vi "ChassisDriveDistanceSmart.vi"(8 "Zero":bool, 9 "DriveRight":dbl, 10 "DriveLeft":dbl) -> ()   [LabVIEW 2014, in "ChassisLib.lvlib"]
uses:
  ChassisLib.lvlib
  ChassisRefs.ctl
  <vilib>/addons/control/pid/pid.llb/PID (DBL).vi
  <vilib>/addons/control/pid/NI_PID_pid.lvlib
panel:
  out "Left":cluster{dbl, "PercentComplete":dbl}(graph)
  out "Right":cluster{dbl, "PercentComplete":dbl}(graph)
  out "PercentComplete":dbl format="%#_13g"
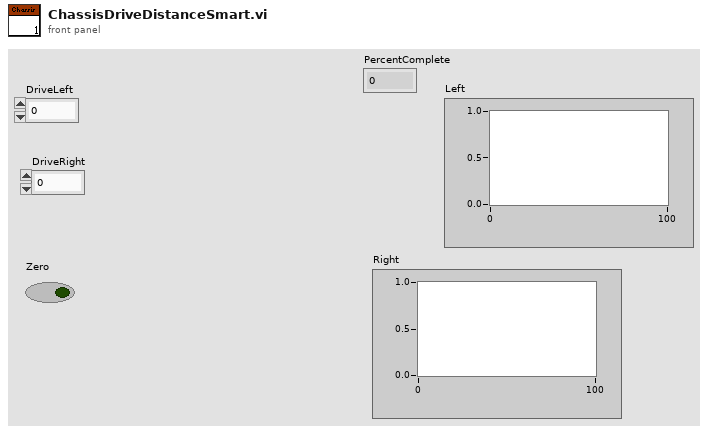
[diagram p1: front panel]
types:
  T1 = typedef "ChassisLib.lvlib/ChassisRefs.ctl" = enum16{"RobotDrive", "Compressor", "DriveEncoderLeft", "DriveEncoderRight", "RioAccel"}
  T2 = typedef "WPI_EncoderDevRef.ctl" = cluster{"DevStatus":errorcluster, "EncoderIndex":T3, "CounterIndex":T4, "DistancePerCount":dbl, "Decoding Type":T5}
  T3 = typedef "FPGA_EncoderIdx.ctl" = enum8{"Enc 0", "Enc 1", "Enc 2", "Enc 3", "Enc 4", "Enc 5", "Enc 6", "Enc 7", "Invalid"}
  T4 = typedef "FPGA_CounterCtrSystemIndex.ctl" = enum8{"Ctr 0", "Ctr 1", "Ctr 2", "Ctr 3", "Ctr 4", "Ctr 5", "Ctr 6", "Ctr 7", "Invalid"}
  T5 = typedef "WPI_EncoderType.ctl" = enum16{"1x", "2x", "4x"}
  T6 = cluster{"proportional gain (Kc)":dbl, "integral time (Ti, min)":dbl, "derivative time (Td, min)":dbl}
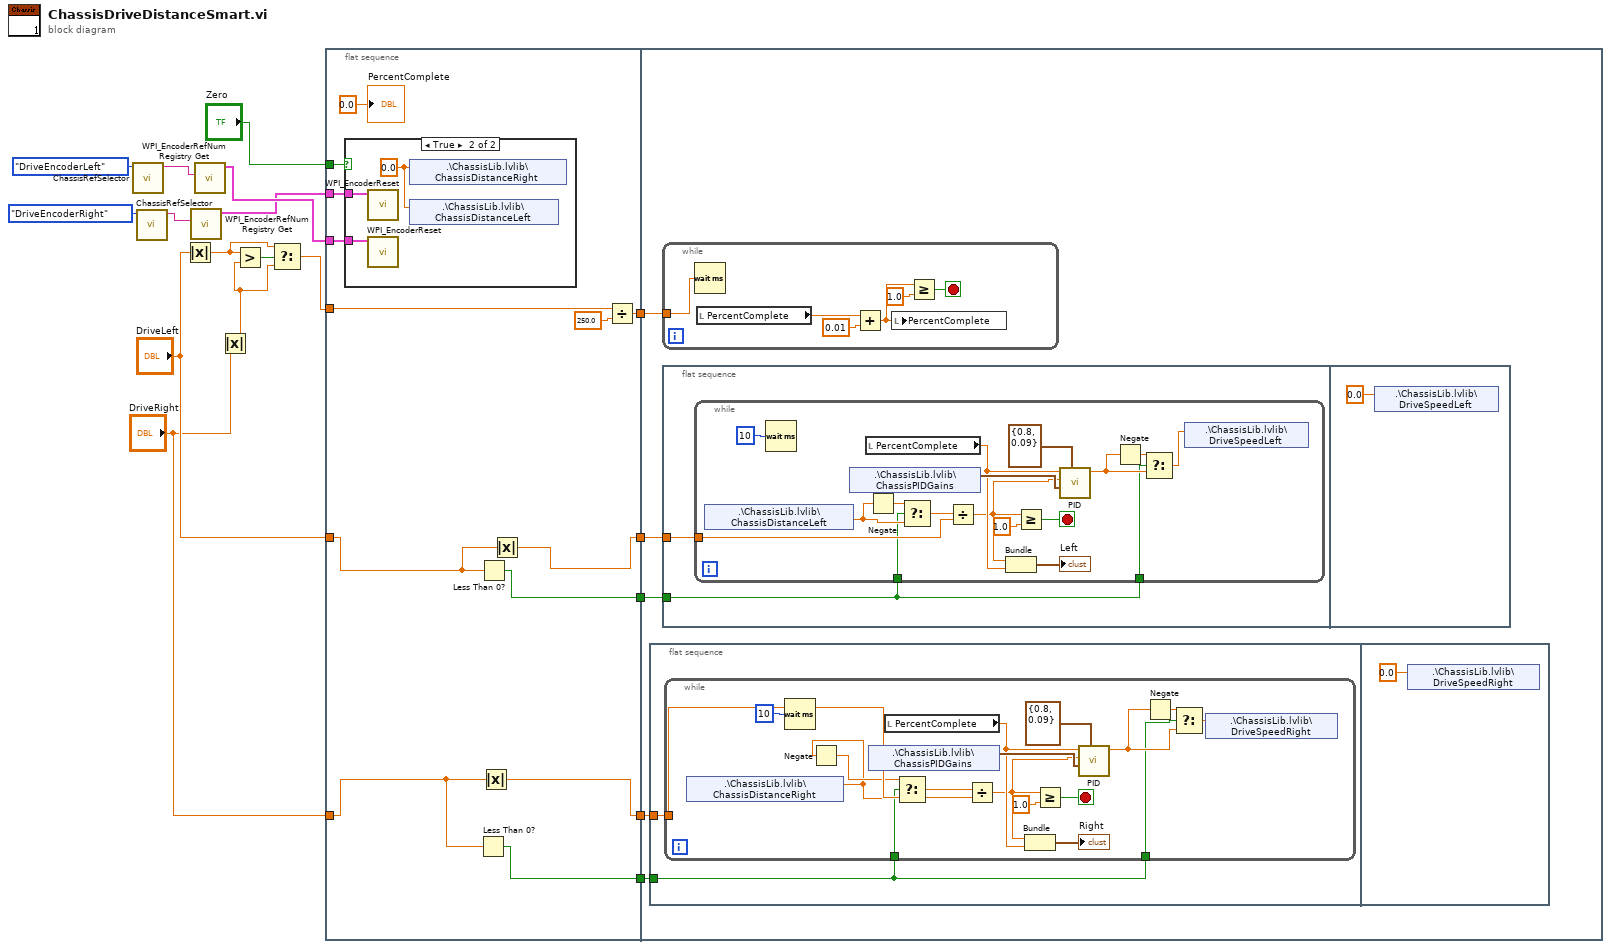
[diagram p0: block diagram]
diagram:
  n1 = call "ChassisRefSelector.vi"("Enum 2"=ChassisRefs."DriveEncoderLeft") -> ("String"=w16:string)  [unwired: 10 in]
  n2 = call "ChassisRefSelector.vi"("Enum 2"=ChassisRefs."DriveEncoderRight") -> ("String"=w15:string)  [unwired: 10 in]
  n3 = Absolute Value(x="DriveLeft") -> (abs(x)=w2:dbl)
  n4 = call <vilib>:"WPI_EncoderRefNum Registry Get.vi"("refnum name"=w15) -> ("EncoderDevRef"=w13:T2)  [unwired: 9 in, 1 out]
  n5 = call <vilib>:"WPI_EncoderRefNum Registry Get.vi"("refnum name"=w16) -> ("EncoderDevRef"=w14:T2)  [unwired: 9 in, 1 out]
  n6 = Absolute Value(x="DriveRight") -> (abs(x)=w1:dbl)
  n7 = Greater?(x=w2, y=w1) -> (0:w12:bool)
  n8 = Select(t=w2, s=w12, f=w1) -> (s? t:f=w11:dbl)
  n9 = flat-sequence {
    tunnel: w14 -> [w31]
    tunnel: w13 -> [w30]
    tunnel: w11 -> [w27]
    tunnel: [w26] -> w10
    tunnel: "DriveLeft" -> [w24]
    tunnel: [w23] -> w8
    tunnel: "DriveRight" -> [w20]
    tunnel: [w21] -> w6
    tunnel: "Zero" -> [w25]
    tunnel: [w22] -> w4
    tunnel: [w19] -> w3
    tunnel: w10 -> [w39]
    tunnel: w8 -> [w38]
    tunnel: w6 -> [w37]
    tunnel: w4 -> [w36]
    tunnel: w3 -> [w35]
    frame #0 {
      n10 = case shown="True" w25 {
        tunnel: w31 -> [_ w34]
        tunnel: w30 -> [_ w33]
        frame False {
        }
        frame True {
          w32 = 0.0 ("ChassisDistanceRight")
          n11 = call <vilib>:"WPI_EncoderReset.vi"("EncoderDevRef"=w33) -> ()  [unwired: 9 in, 2 out]
          n12 = call <vilib>:"WPI_EncoderReset.vi"("EncoderDevRef"=w34) -> ()  [unwired: 9 in, 2 out]
          n13 = shared-variable ".\\ChassisLib.lvlib\\ChassisDistanceRight"(w32) -> ()  [unwired: 1 in, 1 out]
          n14 = shared-variable ".\\ChassisLib.lvlib\\ChassisDistanceLeft"(w32) -> ()  [unwired: 1 in, 1 out]
        }
      }
      n15 = Less Than 0?(x=w20) -> (x < 0?=w19:bool)
      n16 = Less Than 0?(x=w24) -> (x < 0?=w22:bool)
      n17 = Absolute Value(x=w20) -> (abs(x)=w21:dbl)
      n18 = Absolute Value(x=w24) -> (abs(x)=w23:dbl)
      n19 = Divide(x=w27, y=250.0) -> (x/y=w26:dbl)
      "PercentComplete" <- 0.0 ("PercentComplete")
    }
    frame #1 {
      n20 = flat-sequence {
        tunnel: w37 -> [w61]
        tunnel: w35 -> [w60]
        frame #0 {
          n21 = while {
            tunnel: w61 -> [w78]
            tunnel: w60 -> [w66]
            tunnel: w60 -> [w62]
            stop <- w76 stop-if-true
            n22 = shared-variable ".\\ChassisLib.lvlib\\ChassisDistanceRight"() -> (w64:dbl)  [unwired: 1 in, 1 out]
            n23 = Wait (ms)(milliseconds to wait=u32 10) -> ()  [unwired: 1 out]
            n24 = Negate(x=w64) -> (-x=w65:dbl)
            n25 = shared-variable ".\\ChassisLib.lvlib\\ChassisPIDGains"() -> (w73:T6)  [unwired: 1 in, 1 out]
            n26 = local read "PercentComplete"() -> (w72:dbl)
            n27 = Select(t=w65, s=w66, f=w64) -> (s? t:f=w63:dbl)
            n28 = Divide(x=w63, y=w78) -> (x/y=w71:dbl)
            n29 = Bundle(w71, "PercentComplete"=w72) -> (→"Right":cluster{dbl, "PercentComplete":dbl})  [unwired: 1 in]
            n30 = Greater Or Equal?(x=w71, y=1.0) -> (x >= y?=w76:bool)
            n31 = call-poly <vilib>:"PID.vi"("output range"=cluster{"output high":dbl, "output low":dbl} {"output high"=0.8, "output low"=0.09}, "PID gains"=w73, "process variable"=w71, "setpoint"=w72) -> ("output"=w67:dbl)  [unwired: 6 in, 1 out]
            n32 = Negate(x=w67) -> (-x=w69:dbl)
            n33 = Select(t=w69, s=w62, f=w67) -> (s? t:f=w68:dbl)
            n34 = shared-variable ".\\ChassisLib.lvlib\\DriveSpeedRight"(w68) -> ()  [unwired: 1 in, 1 out]
          }
        }
        frame #1 {
          n35 = shared-variable ".\\ChassisLib.lvlib\\DriveSpeedRight"(0.0 ("DriveSpeedRight")) -> ()  [unwired: 1 in, 1 out]
        }
      }
      n36 = while {
        tunnel: w39 -> [w81]
        stop <- w85 stop-if-true
        n37 = Wait (ms)(milliseconds to wait=w81) -> ()  [unwired: 1 out]
        n38 = local read "PercentComplete"() -> (w83:dbl)
        n39 = Add(x=w83, y=0.01) -> (x+y=w82:dbl)
        n40 = local write "PercentComplete"(w82) -> ()
        n41 = Greater Or Equal?(x=w82, y=1.0) -> (x >= y?=w85:bool)
      }
      n42 = flat-sequence {
        tunnel: w38 -> [w41]
        tunnel: w36 -> [w40]
        frame #0 {
          n43 = while {
            tunnel: w41 -> [w58]
            tunnel: w40 -> [w46]
            tunnel: w40 -> [w42]
            stop <- w56 stop-if-true
            n44 = shared-variable ".\\ChassisLib.lvlib\\ChassisDistanceLeft"() -> (w44:dbl)  [unwired: 1 in, 1 out]
            n45 = Wait (ms)(milliseconds to wait=u32 10) -> ()  [unwired: 1 out]
            n46 = shared-variable ".\\ChassisLib.lvlib\\ChassisPIDGains"() -> (w53:T6)  [unwired: 1 in, 1 out]
            n47 = local read "PercentComplete"() -> (w51:dbl)
            n48 = Negate(x=w44) -> (-x=w43:dbl)
            n49 = Select(t=w43, s=w42, f=w44) -> (s? t:f=w45:dbl)
            n50 = Divide(x=w45, y=w58) -> (x/y=w50:dbl)
            n51 = Bundle(w50, "PercentComplete"=w51) -> (→"Left":cluster{dbl, "PercentComplete":dbl})  [unwired: 1 in]
            n52 = Greater Or Equal?(x=w50, y=1.0) -> (x >= y?=w56:bool)
            n53 = call-poly <vilib>:"PID.vi"("output range"=cluster{"output high":dbl, "output low":dbl} {"output high"=0.8, "output low"=0.09}, "PID gains"=w53, "process variable"=w50, "setpoint"=w51) -> ("output"=w47:dbl)  [unwired: 6 in, 1 out]
            n54 = Negate(x=w47) -> (-x=w48:dbl)
            n55 = Select(t=w48, s=w46, f=w47) -> (s? t:f=w49:dbl)
            n56 = shared-variable ".\\ChassisLib.lvlib\\DriveSpeedLeft"(w49) -> ()  [unwired: 1 in, 1 out]
          }
        }
        frame #1 {
          n57 = shared-variable ".\\ChassisLib.lvlib\\DriveSpeedLeft"(0.0 ("DriveSpeedLeft")) -> ()  [unwired: 1 in, 1 out]
        }
      }
    }
  }
